vi "configure.vi"(8 "error in (no error)":errorcluster, 11 "SimulateSerialData in":refnum<class "SimulateSerialData.lvclass">) -> (0 "error out":errorcluster, 3 "SimulateSerialData out":refnum<class "SimulateSerialData.lvclass">)   [LabVIEW 2013, in "SimulateSerialData.lvclass"]
uses:
  SimulateSerialData.lvclass
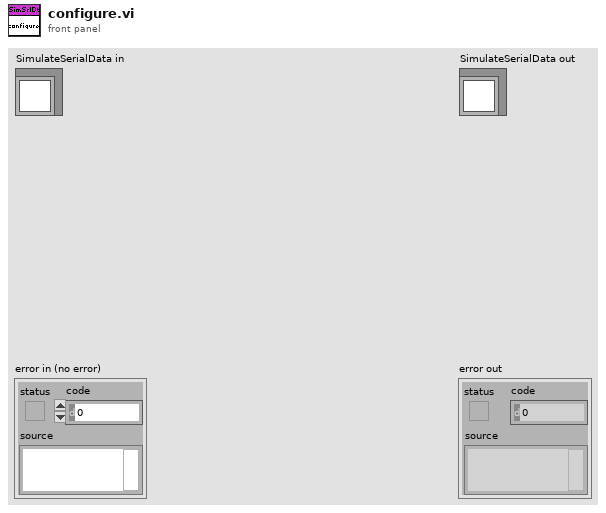
[diagram p1: front panel]
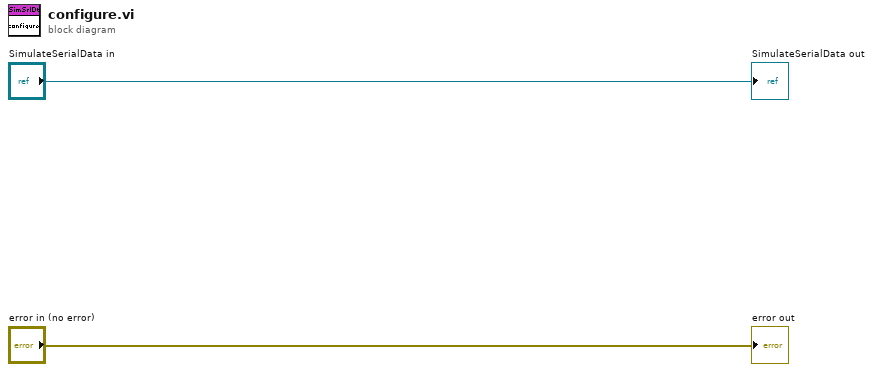
[diagram p0: block diagram]
diagram:
  "error out" <- "error in (no error)"
  "SimulateSerialData out" <- "SimulateSerialData in"
